vi "Get Joystick type.vi"(0 "refnum name":string="My Joystick RefNum", 1 "Pro Joystick":bool) -> (2 "Axes":T3, 3 "Buttons":T2, 4 "Raw Axes":T1, 5 "Raw Buttons":T2)   [LabVIEW 2014]
uses:
  <vilib>/Rock Robotics/WPI/Joystick/WPI_JoystickGetSetRefNum.vi
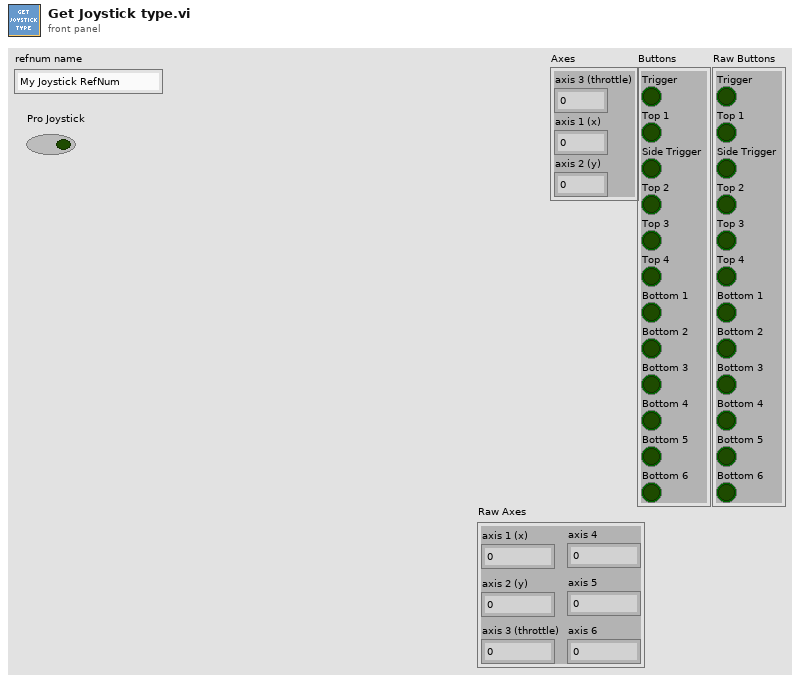
[diagram p1: front panel]
types:
  T1 = cluster{"axis 1 (x)":dbl, "axis 2 (y)":dbl, "axis 3 (throttle)":dbl, "axis 4":dbl, "axis 5":dbl, "axis 6":dbl}
  T2 = cluster{"Trigger":bool, "Top 1":bool, "Side Trigger":bool, "Top 2":bool, "Top 3":bool, "Top 4":bool, "Bottom 1":bool, "Bottom 2":bool, "Bottom 3":bool, "Bottom 4":bool, "Bottom 5":bool, "Bottom 6":bool}
  T3 = cluster{"axis 3 (throttle)":dbl, "axis 1 (x)":dbl, "axis 2 (y)":dbl}
  T4 = typedef "WPI_JoystickDevRef.ctl" = cluster{"Device":T5}
  T5 = typedef "WPI_JoystickDeviceEnum.ctl" = enum16{"USB 0", "USB 1", "USB 2", "USB 3", "USB 4", "USB 5"}
  T6 = cluster{"Button 1":bool, "Button 2":bool, "Button 3":bool, "Button 4":bool, "Button 5":bool, "Button 6":bool, "Button 7":bool, "Button 8":bool, "Button 9":bool, "Button 10":bool, "Button 11":bool, "Button 12":bool}
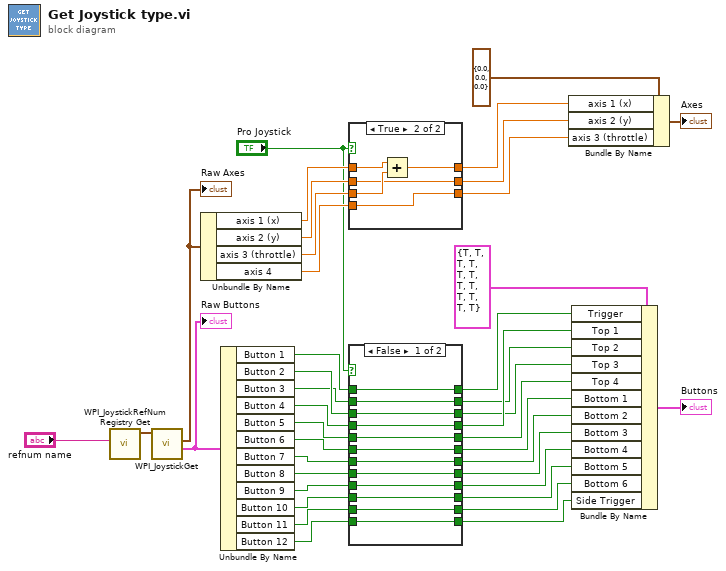
[diagram p0: block diagram]
diagram:
  n1 = call <vilib>:"WPI_JoystickRefNum Registry Get.vi"("refnum name"="refnum name") -> ("JoystickDevRef"=w39:T4)  [unwired: 9 in, 1 out]
  n2 = call <vilib>:"WPI_JoystickGet.vi"("JoystickDevRef"=w39) -> ("Buttons"=w3:T6, "Axes"=w38:T1)  [unwired: 4 in, 1 out]
  "Raw Buttons" <- w3
  "Raw Axes" <- w38
  n3 = Unbundle By Name(w38) -> ("axis 1 (x)"=w37:dbl, "axis 2 (y)"=w36:dbl, "axis 3 (throttle)"=w35:dbl, "axis 4"=w34:dbl)
  n4 = Unbundle By Name(w3) -> ("Button 1"=w29:bool, "Button 2"=w27:bool, "Button 3"=w26:bool, "Button 4"=w25:bool, "Button 5"=w24:bool, "Button 6"=w23:bool, "Button 7"=w22:bool, "Button 8"=w21:bool, "Button 9"=w20:bool, "Button 10"=w19:bool, "Button 11"=w18:bool, "Button 12"=w17:bool)
  n5 = case shown="True" "Pro Joystick" {
    tunnel: w37 -> [w43 w48]
    tunnel: w36 -> [w42 w45]
    tunnel: w35 -> [w41 w47]
    tunnel: w34 -> [_ w44]
    tunnel: [w43 w46] -> w1
    tunnel: [w42 w45] -> w2
    tunnel: [w41 w44] -> w33
    frame False {
    }
    frame True {
      n6 = Add(x=w48, y=w47) -> (x+y=w46:dbl)
    }
  }
  n7 = case shown="False" "Pro Joystick" {
    tunnel: w29 -> [w60 w72]
    tunnel: [w60 w72] -> w28
    tunnel: w27 -> [w51 w71]
    tunnel: w26 -> [w50 w63]
    tunnel: w25 -> [w49 w62]
    tunnel: w24 -> [w52 w64]
    tunnel: w23 -> [w58 w61]
    tunnel: w22 -> [w57 w70]
    tunnel: w21 -> [w56 w69]
    tunnel: w20 -> [w55 w68]
    tunnel: w19 -> [w54 w67]
    tunnel: w18 -> [w53 w66]
    tunnel: w17 -> [w59 w65]
    tunnel: [w49 w64] -> w16
    tunnel: [w50 w63] -> w15
    tunnel: [w51 w62] -> w14
    tunnel: [w52 w61] -> w13
    tunnel: [w58 w70] -> w12
    tunnel: [w57 w69] -> w11
    tunnel: [w56 w68] -> w10
    tunnel: [w55 w67] -> w9
    tunnel: [w54 w66] -> w8
    tunnel: [w53 w65] -> w7
    tunnel: [w59 w71] -> w6
    frame False {
    }
    frame True {
    }
  }
  n8 = Bundle By Name(cluster=T3 {"axis 3 (throttle)"=0.0, "axis 1 (x)"=0.0, "axis 2 (y)"=0.0} ("input cluster"), "axis 1 (x)"=w1, "axis 2 (y)"=w2, "axis 3 (throttle)"=w33) -> (→"Axes":T3)
  n9 = Bundle By Name(cluster=T2 {"Trigger"=TRUE, "Top 1"=TRUE, "Side Trigger"=TRUE, "Top 2"=TRUE, "Top 3"=TRUE, "Top 4"=TRUE, "Bottom 1"=TRUE, "Bottom 2"=TRUE, "Bottom 3"=TRUE, "Bottom 4"=TRUE, "Bottom 5"=TRUE, "Bottom 6"=TRUE} ("input cluster"), "Trigger"=w28, "Top 1"=w16, "Top 2"=w15, "Top 3"=w14, "Top 4"=w13, "Bottom 1"=w12, "Bottom 2"=w11, "Bottom 3"=w10, "Bottom 4"=w9, "Bottom 5"=w8, "Bottom 6"=w7, "Side Trigger"=w6) -> (→"Buttons":T2)
